vi "Circle Geometry Custom Test.vi"(3 "Error In":errorcluster, 4 "Solution VI":path, 5 "User VI":path) -> (0 "Error Out":errorcluster, 2 "Results":T1={"Id"="", "Score"={"Status"=enum."Passed", "cpu_time"=-1, "max_memory"=-1, "style_score"=-1, "score0"="", "score1"="", "score2"="", "score3"="", "score4"="", "score5"=""}})   [LabVIEW 2013]
uses:
  <vilib>/LabVIEW Hacker/VIChallenge/Private/Grader/Type Defs/Grader Result.ctl
  <vilib>/LabVIEW Hacker/VIChallenge/Private/Type Defs/Database/Score.ctl
  <vilib>/LabVIEW Hacker/VIChallenge/Private/Grader/Type Defs/UTF Status.ctl
  <vilib>/LabVIEW Hacker/VIChallenge/VIChallenge.lvlib
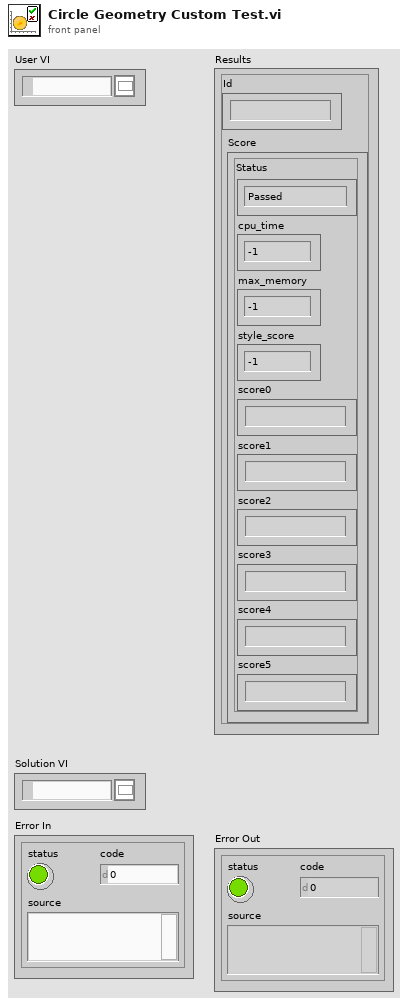
[diagram p1: front panel]
types:
  T1 = typedef "VIChallenge.lvlib/Grader Result.ctl" = cluster{"Id":string, "Score":T2}
  T2 = typedef "VIChallenge.lvlib/Score.ctl" = cluster{"Status":T3, "cpu_time":i32, "max_memory":i32, "style_score":i32, "score0":string, "score1":string, "score2":string, "score3":string, "score4":string, "score5":string}
  T3 = typedef "VIChallenge.lvlib/UTF Status.ctl" = enum16{"Null", "Passed", "Failed", "Error", "Skipped", "Not Processed"}
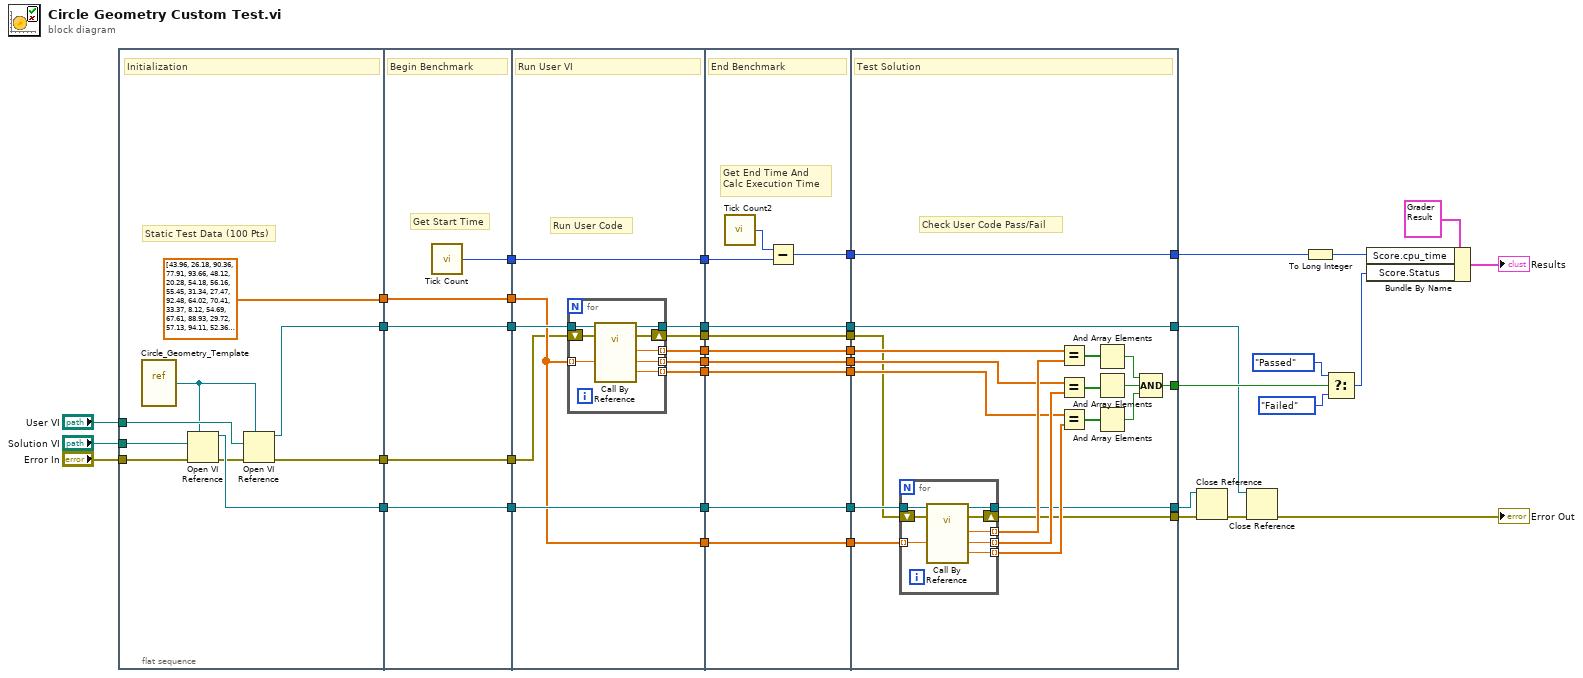
[diagram p0: block diagram]
diagram:
  n1 = flat-sequence {
    tunnel: [dbl[] [43.96, 26.18, 90.36, 77.91, 93.66, 48.12, 20.28, 54.18, 56.16, 55.45, 31.34, 27.47, 92.48, 64.02, 70.41, 33.37, 8.12, 54.69, 67.61, 88.93, 29.72, 57.13, 94.11, 52.36, 16.55, 64.84, 6.34, 70.75, 37.65, 38.91, 77.11, 48.29, 99.06, 64.63, 84.48, 48.81, 21.5, 30.93, 5.17, 90.45, 67.69, 62.11, 19.63, 11.88, 16.1, 33.78, 42.58, 96.17, 83.68, 84.57, 95.98, 44.67, 62.09, 8.32, 76.61, 7.07, 18.33, 48.79, 23.68, 52.32, 62.15, 37.1, 31.49, 22.53, 81.16, 54.53, 81.33, 0.75, 20.9, 81.62, 21.69, 78.94, 12.03, 36.74, 90.57, 75.51, 54.89, 91.2, 63.32, 83.92, 93.27, 38.68, 82.82, 9.85, 59.76, 36.3, 6.29, 64.4, 23.18, 8.01, 63.29, 58.89, 52.0, 74.4, 41.31, 43.39, 22.09, 84.27, 82.68, 30.12] ("x/y")] -> w40
    tunnel: "User VI" -> [w49]
    tunnel: [w48] -> w38
    tunnel: "Solution VI" -> [w47]
    tunnel: [w46] -> w26
    tunnel: "Error In" -> [w44]
    tunnel: [w42] -> w14
    tunnel: [w55] -> w41
    tunnel: w40 -> [w55]
    tunnel: w38 -> [w54]
    tunnel: [w54] -> w37
    tunnel: [w53] -> w31
    tunnel: [w52] -> w27
    tunnel: w26 -> [w52]
    tunnel: w14 -> [w51]
    tunnel: [w51] -> w13
    tunnel: w41 -> [w59]
    tunnel: w37 -> [w65]
    tunnel: [w64] -> w36
    tunnel: [w63] -> w35
    tunnel: [w62] -> w34
    tunnel: [w61] -> w32
    tunnel: w31 -> [w61]
    tunnel: [w60] -> w28
    tunnel: w27 -> [w60]
    tunnel: [w59] -> w25
    tunnel: w13 -> [w58]
    tunnel: [w57] -> w11
    tunnel: [w56] -> w5
    tunnel: w36 -> [w79]
    tunnel: w35 -> [w78]
    tunnel: w34 -> [w77]
    tunnel: w32 -> [w83]
    tunnel: [w82] -> w30
    tunnel: [w81] -> w29
    tunnel: w28 -> [w81]
    tunnel: w25 -> [w80]
    tunnel: [w80] -> w24
    tunnel: [w79] -> w23
    tunnel: [w78] -> w22
    tunnel: [w77] -> w21
    tunnel: [w75] -> w12
    tunnel: w11 -> [w75]
    tunnel: [w74] -> w6
    tunnel: w5 -> [w74]
    tunnel: w30 -> [w103]
    tunnel: [w103] -> w1
    tunnel: w29 -> [w102]
    tunnel: w24 -> [w101]
    tunnel: w23 -> [w100]
    tunnel: w22 -> [w98]
    tunnel: w21 -> [w95]
    tunnel: [w88] -> w19
    tunnel: w12 -> [w87]
    tunnel: [w86] -> w10
    tunnel: [w85] -> w8
    tunnel: [w84] -> w7
    tunnel: w6 -> [w84]
    frame #0 {
      # "Static Test Data (100 Pts)"
      # "Initialization"
      n2 = vi-ref <vilib>:"Circle_Geometry_Template.vi"() -> (w45:refnum<vi>)
      n3 = Open VI Reference(type specifier VI Refnum (for type only)=w45, vi path=w47, error in (no error)=w44) -> (vi reference=w46:refnum<vi>, error out=w43:errorcluster)  [unwired: 3 in]
      n4 = Open VI Reference(type specifier VI Refnum (for type only)=w45, vi path=w49, error in (no error)=w43) -> (vi reference=w48:refnum<vi>, error out=w42:errorcluster)  [unwired: 3 in]
    }
    frame #1 {
      # "Get Start Time"
      # "Begin Benchmark"
      n5 = call "Tick Count"() -> ("Tick Count(uSec)"=w53:u32)
    }
    frame #2 {
      # "Run User Code"
      # "Run User VI"
      n6 = for {
        tunnel: w65 -> [w73]
        tunnel: w59 -> [w72] mode=indexing
        tunnel: [w71] -> w64 mode=indexing
        tunnel: [w70] -> w63 mode=indexing
        tunnel: [w69] -> w62 mode=indexing
        shift-right: [w67] -> w57
        shift-left: w58 -> [w68]
        tunnel: [w66] -> w56
        n7 = call-by-ref "?"(reference=w73, error in=w68, "Radius"=w72) -> (reference out=w66:refnum<vi>, error out=w67:errorcluster, "Area"=w69:dbl, "Circumference"=w70:dbl, "Diameter"=w71:dbl)  [unwired: 2 in]
      }
    }
    frame #3 {
      # "Get End Time And \nCalc Execution Time"
      # "End Benchmark"
      n8 = call "Tick Count2"() -> ("Tick Count(uSec)"=w76:u32)
      n9 = Subtract(x=w76, y=w83) -> (x-y=w82:u32)
    }
    frame #4 {
      # "Check User Code Pass/Fail"
      # "Test Solution"
      n10 = for {
        tunnel: w102 -> [w111]
        tunnel: w101 -> [w110] mode=indexing
        tunnel: [w109] -> w99 mode=indexing
        tunnel: [w108] -> w97 mode=indexing
        tunnel: [w107] -> w96 mode=indexing
        shift-right: [w105] -> w86
        shift-left: w87 -> [w106]
        tunnel: [w104] -> w85
        n11 = call-by-ref "?"(reference=w111, error in=w106, "Radius"=w110) -> (reference out=w104:refnum<vi>, error out=w105:errorcluster, "Area"=w107:dbl, "Circumference"=w108:dbl, "Diameter"=w109:dbl)  [unwired: 2 in]
      }
      n12 = Equal?(x=w100, y=w99) -> (x = y?=w94:bool[])
      n13 = Equal?(x=w98, y=w97) -> (x = y?=w93:bool[])
      n14 = Equal?(x=w95, y=w96) -> (x = y?=w92:bool[])
      n15 = And Array Elements(Boolean array=w94) -> (logical AND=w91:bool)
      n16 = And Array Elements(Boolean array=w93) -> (logical AND=w90:bool)
      n17 = And Array Elements(Boolean array=w92) -> (logical AND=w89:bool)
      n18 = Compound Arithmetic op=AND(w91, w90, w89) -> (w88:bool)
    }
  }
  n19 = Close Reference(reference=w8, error in (no error)=w10) -> (error out=w9:errorcluster)
  n20 = Close Reference(reference=w7, error in (no error)=w9) -> (error out=→"Error Out":errorcluster)
  n21 = To Long Integer(number=w1) -> (32bit integer=w2:i32)
  n22 = Select(t=UTF_Status."Passed" ("Score.Status"), s=w19, f=UTF_Status."Failed" ("Score.Status")) -> (s? t:f=w4:T3)
  n23 = Bundle By Name(cluster=T1 {"Id"="", "Score"={"Status"=enum."Passed", "cpu_time"=-1, "max_memory"=-1, "style_score"=-1, "score0"="", "score1"="", "score2"="", "score3"="", "score4"="", "score5"=""}} ("Grader Result (Error)"), "Score.cpu_time"=w2, "Score.Status"=w4) -> (→"Results":T1)
